vi "FABR-Init Frequency.vi"(0 "Stimulus":T3={"Destination"="", "Rep rate (/sec)"=30.0, "Alternate Polarity"=FALSE, "Duration (ms)"=20.0, "Ramp (ms)"=80.0, "Fs (Hz)"=5.0, "Frame size (s)"=0.0}, 5 "Sequence":T1={"Freq"={"Expression"="", "Skip"=80}, "Level"={"Start (dB)"=20, "Stop (dB)"=80, "Step (dB)"=5}, "Order"=enum."Interleaved"} {"Level"."Start (dB)" step=5}, 7 "Data folder":path, 11 "error in (no error)":errorcluster) -> (6 "Frequency (kHz)":dbl[](array[numeric]), 8 "Ceilings":dbl[](array[numeric]), 10 "Order":i32[](array[numeric]), 15 "error out":errorcluster)   [LabVIEW 2020]
uses:
  Typedefs/FABR-Stimulus.ctl
  Typedefs/FABR-Sequence.ctl
  Typedefs/FABR-Order.ctl
  4456a615-68eb-4342-ae34-4d8b9cb19531.vi
  epl-vi-lib/Utility VIs/Math VIs/LinSpace (x0-dx-npts).vi
  c8e3877d-62d9-4c57-9062-2c2c28311255.vi
  1f6a5090-8e97-4df4-9b62-a93c2d4c0423.vi
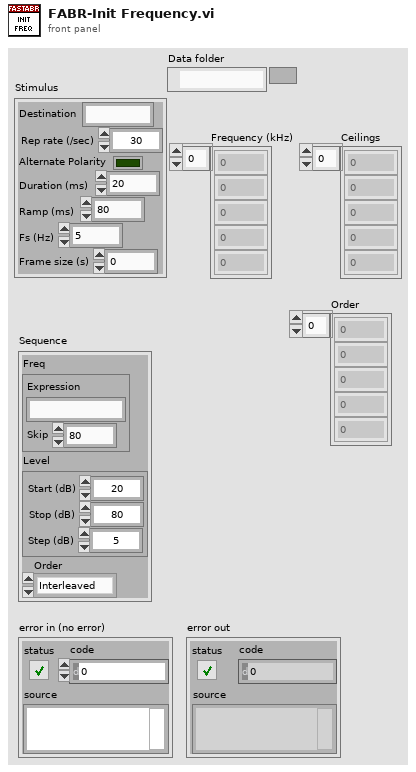
[diagram p1: front panel]
types:
  T1 = typedef "FABR-Sequence.ctl" = cluster{"Freq":cluster{"Expression":string, "Skip":i32}, "Level":cluster{"Start (dB)":i32, "Stop (dB)":i32, "Step (dB)":i32}, "Order":T2}
  T2 = typedef "FABR-Order.ctl" = enum16{"Interleaved", "Step level"}
  T3 = typedef "FABR-Stimulus.ctl" = cluster{"Destination":string, "Rep rate (/sec)":dbl, "Alternate Polarity":bool, "Duration (ms)":dbl, "Ramp (ms)":dbl, "Fs (Hz)":dbl, "Frame size (s)":dbl}
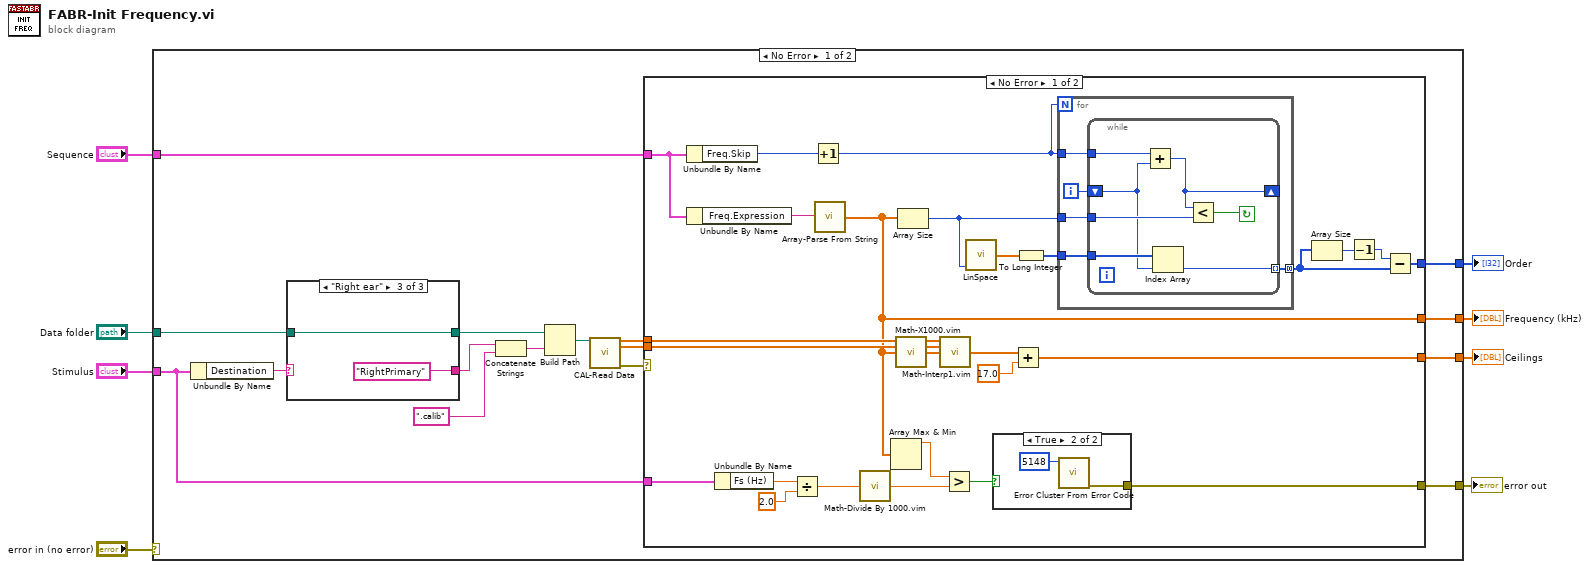
[diagram p0: block diagram]
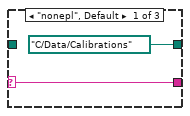
[diagram p4: hidden frame]
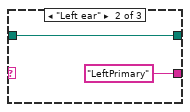
[diagram p5: hidden frame]
diagram:
  n1 = case shown="No Error" "error in (no error)" {
    selector: "error in (no error)" -> [_ w72]
    tunnel: "Sequence" -> [w24 _]
    tunnel: [w23 w72] -> w7
    tunnel: "Stimulus" -> [w22 _]
    tunnel: "Data folder" -> [w21 _]
    tunnel: [w10 _] -> w3
    tunnel: [w11 _] -> w2
    tunnel: [w9 _] -> w1
    frame No Error {
      n2 = Unbundle By Name(w22) -> ("Destination"=w20:string)
      n3 = case shown="\"Right ear\"" w20 {
        selector: w20 -> [w66 _ _]
        tunnel: [w66 "LeftPrimary" "RightPrimary"] -> w18
        tunnel: [path "C:/Data/Calibrations" ("Data folder") w68 w70] -> w19
        tunnel: w21 -> [_ w68 w70]
        frame "nonepl", Default {
        }
        frame "Left ear" {
        }
        frame "Right ear" {
        }
      }
      n4 = Concatenate Strings(w18, ".calib") -> (w13:string)
      n5 = Build Path(base path=w19, name or relative path=w13) -> (appended path=w17:path)
      n6 = call "CAL-Read Data.vi"("user path"=w17) -> ("Frequency (Hz)"=w16:dbl[], "Mag"=w15:dbl[], "error out"=w14:errorcluster)  [unwired: 10 in, 2 out]
      n7 = case shown="No Error" w14 {
        selector: w14 -> [_ w65]
        tunnel: w24 -> [w28 _]
        tunnel: [w44 w65] -> w23
        tunnel: w22 -> [w42 _]
        tunnel: w16 -> [w41 _]
        tunnel: w15 -> [w40 _]
        tunnel: [w34 _] -> w11
        tunnel: [w26 _] -> w10
        tunnel: [w31 _] -> w9
        frame No Error {
          n8 = Unbundle By Name(w28) -> ("Freq.Skip"=w50:i32)
          n9 = Unbundle By Name(w28) -> ("Freq.Expression"=w27:string)
          n10 = Unbundle By Name(w42) -> ("Fs (Hz)"=w49:dbl)
          n11 = Divide(x=w49, y=2.0) -> (x/y=w47:dbl)
          n12 = Increment(x=w50) -> (x+1=w25:i32)
          n13 = call "Array-Parse From String.vi"("String"=w27) -> ("Array"=w26:dbl[])  [unwired: 13 in, 1 out]
          n14 = call "Math-Divide By 1000.vim"("X"=w47) -> ("1000X"=w43:dbl)
          n15 = Array Max & Min(array=w26) -> (max value=w46:dbl)  [unwired: 3 out]
          n16 = call "Math-X1000.vim"("X"=w26) -> ("1000X"=w33:dbl[])
          n17 = Array Size(array=w26) -> (size(s)=w37:i32)
          n18 = call "Math-Interp1.vim"("X"=w41, "Y"=w40, "U"=w33) -> ("V"=w39:dbl[])  [unwired: 12 in]
          n19 = Greater?(x=w46, y=w43) -> (0:w45:bool)
          n20 = call-poly "LinSpace.vi"("npts"=w37) -> ("Array"=w36:dbl[])  [unwired: 3 in, 1 out]
          n21 = case shown="True" w45 {
            tunnel: [_ w52] -> w44
            frame False {
            }
            frame True {
              n22 = call <vilib>:"Error Cluster From Error Code.vi"("error code (0)"=5148) -> ("error out"=w52:errorcluster)  [unwired: 8 in]
            }
          }
          n23 = Add(x=w39, y=17.0 ("Default (NaN)")) -> (x+y=w34:dbl[])
          n24 = To Long Integer(number=w36) -> (32bit integer=w35:i32[])
          n25 = for {
            N: w25 -> [_]
            tunnel: w25 -> [w57]
            tunnel: w37 -> [w55]
            tunnel: w35 -> [w54]
            tunnel: [w53] -> w32 mode=concatenating
            i -> [w56]
            n26 = while {
              tunnel: w57 -> [w64]
              shift-right: [w63] -> _
              shift-left: w56 -> [w59]
              tunnel: w55 -> [w62]
              tunnel: w54 -> [w60]
              tunnel: [w58] -> w53 mode=indexing
              stop <- w61 continue-if-true
              n27 = Add(x=w64, y=w59) -> (x+y=w63:i32)
              n28 = Index Array(array=w60, index=w59) -> (element=w58:i32)
              n29 = Less?(x=w63, y=w62) -> (x < y?=w61:bool)
            }
          }
          n30 = Array Size(array=w32) -> (size(s)=w30:i32)
          n31 = Decrement(x=w30) -> (x-1=w29:i32)
          n32 = Subtract(x=w29, y=w32) -> (x-y=w31:i32[])
        }
        frame Error {
        }
      }
    }
    frame Error {
    }
  }
  "error out" <- w7
  "Frequency (kHz)" <- w3
  "Ceilings" <- w2
  "Order" <- w1
